vi "EfcoBackendService.vi"(7 "LabVIEW Web Service Request":refnum<class "Web Request.lvclass">, 9 "minimumTolerance":dbl, 10 "maximumTolerance":dbl, 11 "targetPressure":dbl) -> (2 "value":string, 3 "maximumPressure":dbl format="%0.2f")   [LabVIEW 2015]
uses:
  <vilib>/wsapi/Web Request.lvclass
  Control test 1.ctl
  <vilib>/Waveform/WDTOps.llb/WDT Append Waveforms DBL.vi
panel:
  out "target_pr":dbl
  in  "stop (F)":bool
  out "data":T1
  out "current pr":dbl
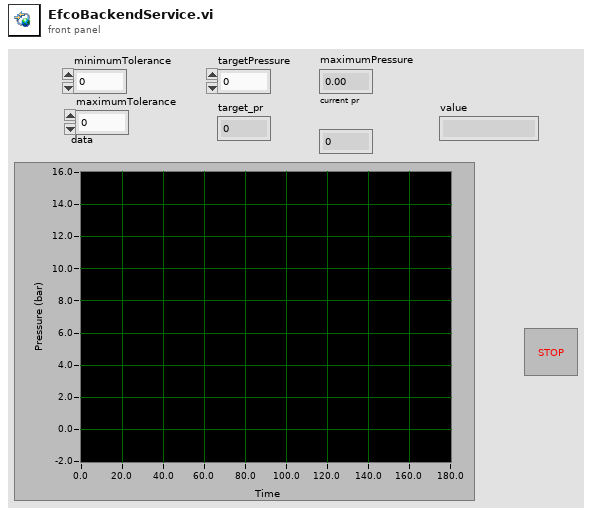
[diagram p1: front panel]
types:
  T1 = typedef "Control test 1.ctl" = dynamicdata
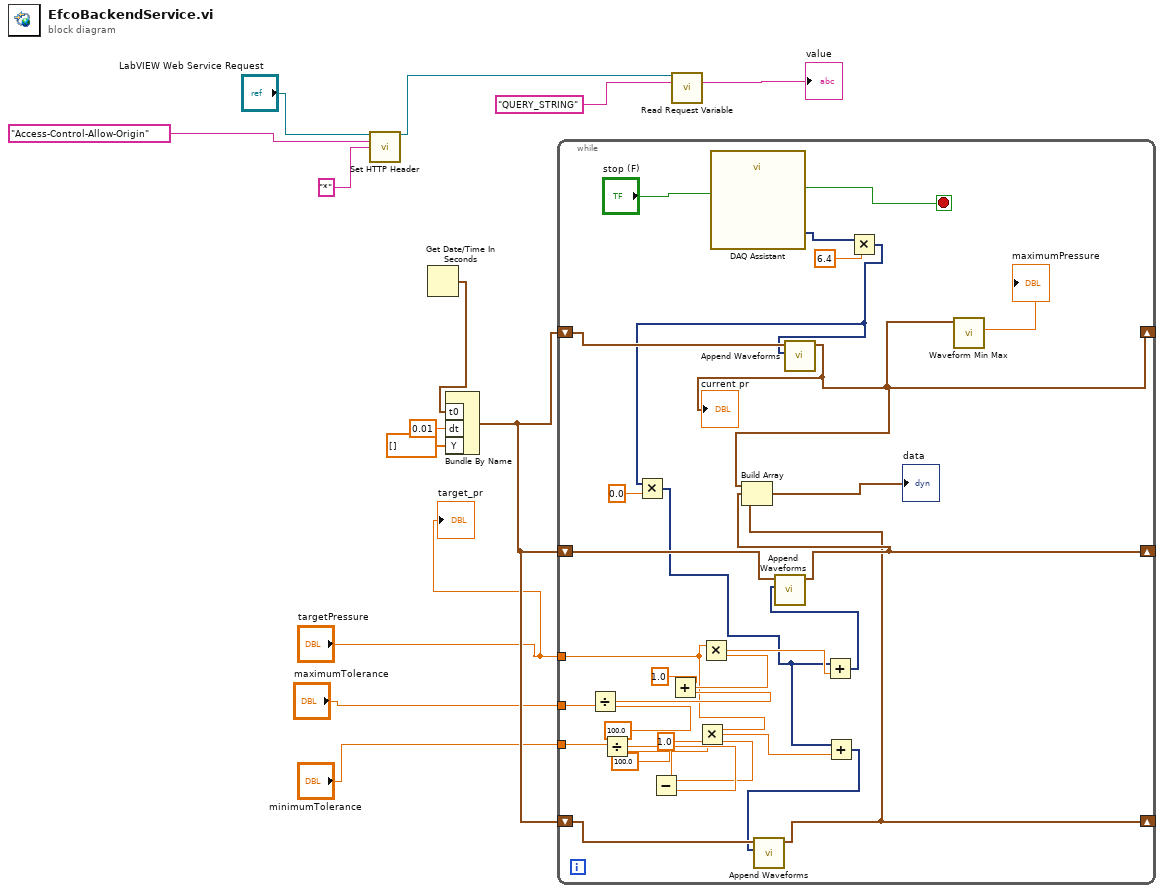
[diagram p0: block diagram]
diagram:
  n1 = call <vilib>:"Set HTTP Header.vi"("LabVIEW Web Service Request"="LabVIEW Web Service Request", "header"="Access-Control-Allow-Origin", "header value"="*") -> ("LabVIEW Web Service Request out"=w1:refnum<class "Web Request.lvclass">)  [unwired: 11 in, 1 out]
  n2 = Get Date/Time In Seconds() -> (seconds since 1Jan1904=w9:timestamp)
  n3 = Bundle By Name("t0"=w9, "dt"=0.01, "Y"=dbl[] []) -> (w8:waveform(dbl))  [unwired: 1 in]
  n4 = while {
    shift-right: [w15] -> _
    shift-left: w8 -> [w18]
    shift-right: [w39] -> _
    shift-left: w8 -> [w40]
    tunnel: "maximumTolerance" -> [w38]
    tunnel: "minimumTolerance" -> [w36]
    tunnel: "targetPressure" -> [w28]
    shift-right: [w23] -> _
    shift-left: w8 -> [w24]
    stop <- w42 stop-if-true
    n5 = Divide(x=w38, y=100.0) -> (x/y=w33:dbl)
    n6 = Divide(x=w36, y=100.0) -> (x/y=w32:dbl)
    n7 = Subtract(x=1.0, y=w32) -> (x-y=w30:dbl)
    n8 = Add(x=1.0, y=w33) -> (x+y=w29:dbl)
    n9 = Multiply(x=w28, y=w30) -> (x*y=w21:dbl)
    n10 = Multiply(x=w28, y=w29) -> (x*y=w26:dbl)
    n11 = call "DAQ Assistant"("stop (F)"="stop (F)") -> ("data"=w19:dynamicdata, "stopped"=w42:bool)  [unwired: 15 in, 2 out]
    n12 = Multiply(x=w19, y=6.4) -> (x*y=w16:dynamicdata)
    n13 = Multiply(x=w16, y=0.0) -> (x*y=w22:dynamicdata)
    n14 = call-poly <vilib>:"Append Waveforms.vi"("waveform B"=w16, "waveform A"=w18) -> ("waveform out"=w15:waveform(dbl))  [unwired: 8 in, 1 out]
    "current pr" <- w15
    n15 = Add(x=w22, y=w26) -> (x+y=w25:dynamicdata)
    n16 = call-poly <vilib>:"Append Waveforms.vi"("waveform B"=w25, "waveform A"=w40) -> ("waveform out"=w39:waveform(dbl))  [unwired: 8 in, 1 out]
    n17 = Add(x=w22, y=w21) -> (x+y=w20:dynamicdata)
    n18 = call-poly <vilib>:"Append Waveforms.vi"("waveform B"=w20, "waveform A"=w24) -> ("waveform out"=w23:waveform(dbl))  [unwired: 8 in, 1 out]
    n19 = Build Array(w15, w39, w23) -> (→"data":waveform(dbl)[])
    n20 = call <vilib>:"Waveform Min Max.vi"("waveform in"=w15) -> ("Y max"=→"maximumPressure":dbl)  [unwired: 5 in, 5 out]
  }
  n21 = call <vilib>:"Read Request Variable.vi"("LabVIEW Web Service Request"=w1, "variable name"="QUERY_STRING") -> ("value"=→"value":string)  [unwired: 11 in, 2 out]
  "target_pr" <- "targetPressure"
